vi "Class Loading Result.vi"(0 "Class Loader Interfaces in":refnum<class "Class Loader Interfaces.lvclass">, 5 "Classes Map":T1, 7 "Class Array":refnum<class>[](array[class]), 9 "Class Names":string[](array[string]), 11 "error in (no error)":errorcluster) -> (4 "Class Loader Interfaces out":refnum<class "Class Loader Interfaces.lvclass">, 15 "error out":errorcluster)   [LabVIEW 2023, in "Class Loader.lvlib" / "Class Loader Interfaces.lvclass"]
uses:
  Class Loader Interfaces.lvclass
  Class Loader/Classes Map.ctl
  Class Loader/Class Loader.lvclass
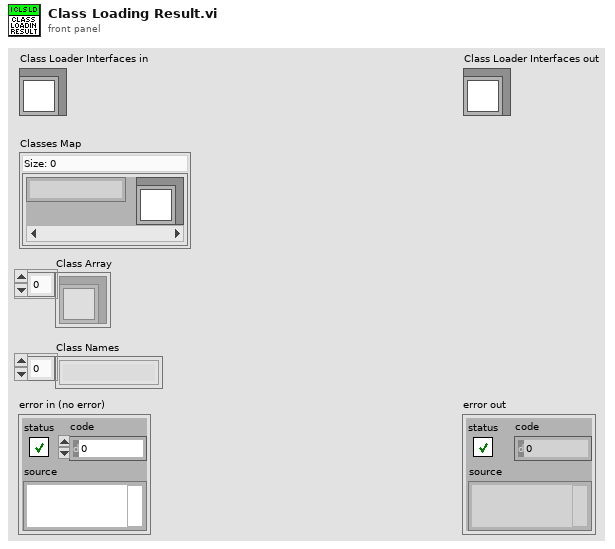
[diagram p1: front panel]
types:
  T1 = typedef "Class Loader.lvlib/Class Loader.lvclass/Classes Map.ctl" = map{string, refnum<class>}
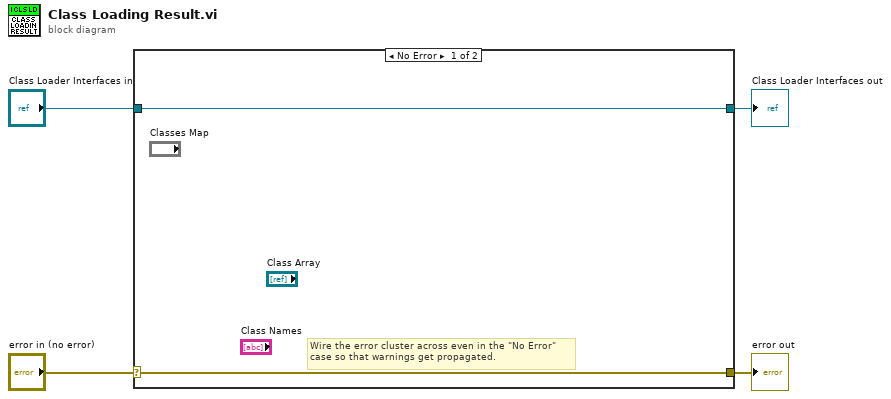
[diagram p0: block diagram]
diagram:
  n1 = case shown="No Error" "error in (no error)" {
    selector: "error in (no error)" -> [w5 w8]
    tunnel: [w5 w8] -> w3
    tunnel: [w6 w7] -> w1
    tunnel: "Class Loader Interfaces in" -> [w6 w7]
    frame No Error {
      # "Wire the error cluster across even in the \"No Error\"\ncase so that warnings get propagated."
    }
    frame Error {
    }
  }
  "error out" <- w3
  "Class Loader Interfaces out" <- w1
